vi "ODE-Disease.vi"() -> ()   [LabVIEW 2023]
doc: "This example demonstrates how to use the polymorphic ODE solver in both Formula Sting mode and VI mode. Note that VI mode allows the user to set the values of constants via front panel controls, and the formula is implemented as a call by reference to another VI."
uses:
  <vilib>/Simulation/Utility/Implementation/Shared/SIM Diagram Parameters.ctl
  <vilib>/Simulation/Implementation/Shared/SIM Continuous Solvers.ctl
  <vilib>/gmath/ode.llb/ODE Solver formula string.vi
  <vilib>/gmath/ode.llb/ODE Solver main.vi
  <vilib>/gmath/NI_Gmath.lvlib
panel:
  out "Population vs. Time":cluster{"times":dbl[], dbl[]}[](graph)
  in  "Stop":bool
  in  "Constants":cluster{"k1":dbl, "k2":dbl}={"k1"=0.2, "k2"=0.7}
  in  "Initial Conditions for  variables (s, i, r)":dbl[](array[numeric])=[50.0, 10.0, 0.0]
  in  "Formula String Parameters":T1={"ODE Right Hand Side"=["-k1*s*i", "-k2*i + k1*s*i", "k2*i"], "X (name of variables)"=["s", "i", "r"], "time"="t"}
  # "Overview: This example demonstrates how to use the polymorphic ODE solver in both Formula Sting mode and VI  mode for the Communicable Diseases model.\nRequirements: LabVIEW Full Development System\nInstructions: \n1. Run the VI.\n2. Modify the input parameters of the ODE solver(s).\n3. Click Stop to stop the VI."
  # "This example demonstrates how to use the polymorphic ODE solver in both Formula Sting mode and VI  mode for the Communicable Diseases model:\n\nds/dt =-k1si\ndi/dt = -k2i + k1si\ndr/dt = k2i\n\nwhere s(t), i(t), r(t) are the populations of those susceptible to, infected by, and recovered from the disease, respectively.  k1 is the infection rate, and k2 is the removal rate."
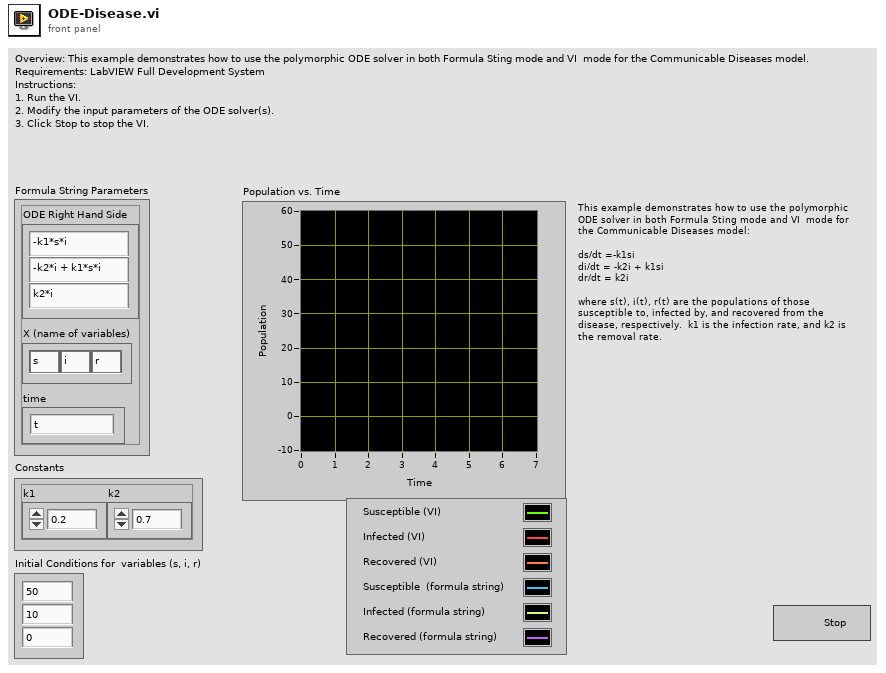
[diagram p1: front panel]
types:
  T1 = cluster{"ODE Right Hand Side":string[], "X (name of variables)":string[], "time":string}
  T2 = typedef "SIM Diagram Parameters.ctl" = cluster{"Initial Time":dbl, "Final Time":dbl, "Time Step":dbl, "Absolute Tolerance":dbl, "Relative Tolerance":dbl, "Continuous Solver":T3, "Discrete Time Step":dbl, "Minimum Time Step":dbl, "Maximum Time Step":dbl, "Initial Time Step":dbl}
  T3 = typedef "SIM Continuous Solvers.ctl" = enum16{"Runge-Kutta 1 (Euler)", "Runge-Kutta 2", "Runge-Kutta 3", "Runge-Kutta 4", "Runge-Kutta 23 (variable)", "Runge-Kutta 45 (variable)", "BDF (variable)", "Adams-Moulton (variable)", "Rosenbrock (variable)", "Discrete States Only"}
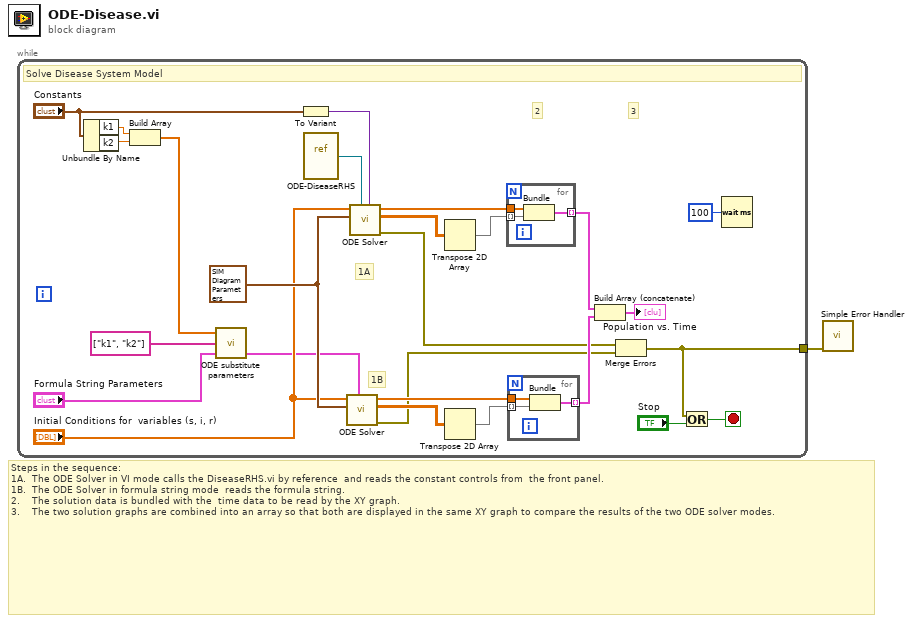
[diagram p0: block diagram]
diagram:
  # "Steps in the sequence:\n1A.  The ODE Solver in VI mode calls the DiseaseRHS.vi by reference  and reads the constant controls from  the front panel.\n1B.  The ODE Solver in formula string mode  reads the formula string.\n2.    The solution data is bundled with the  time data to be read by the XY graph.\n3.    The two solution graphs are combined into an array so that both are displayed in the same XY graph to compare the results of the two ODE solver modes."
  n1 = while {
    tunnel: [w2] -> w1
    stop <- w5 stop-if-true
    w23 = T2 {"Initial Time"=0.0, "Final Time"=7.0, "Time Step"=0.1, "Absolute Tolerance"=0.001, "Relative Tolerance"=1e-06, "Continuous Solver"=enum."Adams-Moulton (variable)", "Discrete Time Step"=2.0, "Minimum Time Step"=1e-06, "Maximum Time Step"=1.0, "Initial Time Step"=0.01} ("Simulation Parameters")
    # "3"
    # "1B"
    # "2"
    # "1A"
    # "Solve Disease System Model"
    n2 = Unbundle By Name("Constants") -> ("k1"=w10:dbl, "k2"=w9:dbl)
    n3 = Build Array(w10, w9) -> (w8:dbl[])
    n4 = call "ODE substitute parameters.vi"("Formula String Parameters"="Formula String Parameters", "parameters"=string[] ["k1", "k2"], "values"=w8) -> ("Formula String Parameters with substitutions"=w12:T1)  [unwired: 2 out]
    n5 = To Variant(anything="Constants") -> (Variant=w17:variant)
    n6 = vi-ref "ODE-DiseaseRHS.vi"() -> ("vi reference"=w27:refnum<vi>)
    n7 = call-poly <vilib>:"ODE Solver.vi"("ODE RHS"=w12, "simulation parameters"=w23, "x0"="Initial Conditions for  variables (s, i, r)") -> ("error out"=w4:errorcluster, "outputs"=w6:dbl[][], "times"=w22:dbl[])  [unwired: 1 in, 5 out]
    n8 = call-poly <vilib>:"ODE Solver.vi"("data"=w17, "ODE F(X,t)"=w27, "simulation parameters"=w23, "x0"="Initial Conditions for  variables (s, i, r)") -> ("error out"=w3:errorcluster, "outputs"=w24:dbl[][], "times"=w25:dbl[])  [unwired: 1 in, 4 out]
    n9 = Transpose 2D Array(2D array=w24) -> (transposed array=w26:dbl[][])
    n10 = Transpose 2D Array(2D array=w6) -> (transposed array=w20:dbl[][])
    n11 = for {
      tunnel: w26 -> [w33] mode=indexing
      tunnel: w25 -> [w32]
      tunnel: [w31] -> w19 mode=indexing
      n12 = Bundle("times"=w32, w33) -> (w31:cluster{"times":dbl[], dbl[]})  [unwired: 1 out]
    }
    n13 = for {
      tunnel: w20 -> [w30] mode=indexing
      tunnel: w22 -> [w29]
      tunnel: [w28] -> w21 mode=indexing
      n14 = Bundle("times"=w29, w30) -> (w28:cluster{"times":dbl[], dbl[]})  [unwired: 1 out]
    }
    n15 = Build Array (concatenate)(w19, w21) -> (→"Population vs. Time":cluster{"times":dbl[], dbl[]}[])
    n16 = Merge Errors(w3, w4) -> (w2:errorcluster)
    n17 = Or(x=w2, y="Stop") -> (x .or. y?=w5:bool)
    n18 = Wait (ms)(milliseconds to wait=u32 100 ("millisecond multiple")) -> ()  [unwired: 1 out]
  }
  n19 = call <vilib>:"Simple Error Handler.vi"("error in (no error)"=w1) -> ()  [unwired: 4 in, 5 out]
